vi "Processed_Bytes_To_CM_Packet.vi"(3 "error in (no error)":errorcluster, 4 "Processed Byte":u8[](array[numeric]), 5 "CM Packet In":T1) -> (0 "error out":errorcluster, 1 "CM Params":T5, 2 "CM Packet Out":T1)   [LabVIEW 2017]
uses:
  Controls/Packet/Packet.ctl
  Controls/Packet/Packet_Direction.ctl
  Controls/Packet/Packet_Type.ctl
  Controls/Packet/Packet_Priority.ctl
  Controls/Control Packets/CM_Param.ctl
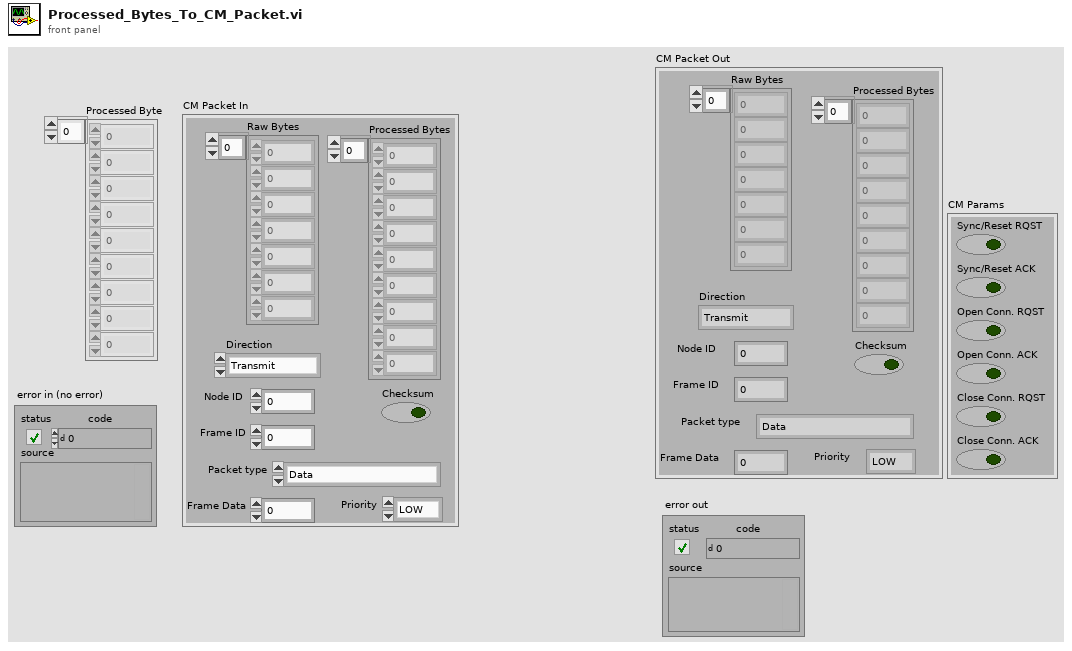
[diagram p1: front panel]
types:
  T1 = typedef "Packet.ctl" = cluster{"Raw Bytes":u8[], "Checksum":bool, "Direction":T2, "Processed Bytes":u8[], "Node ID":u8, "Packet type":T3, "Frame Data":u32, "Priority":T4, "Frame ID":u8}
  T2 = typedef "Packet_Direction.ctl" = enum16{"Transmit", "Receive", "Bidirectional"}
  T3 = typedef "Packet_Type.ctl" = enum16{"Data", "Connection Management", "Remote Request", "Error/Status"}
  T4 = typedef "Packet_Priority.ctl" = enum16{"LOW", "HIGH"}
  T5 = typedef "CM_Param.ctl" = cluster{"Sync/Reset RQST":bool, "Sync/Reset ACK":bool, "Open Conn. RQST":bool, "Open Conn. ACK":bool, "Close Conn. RQST":bool, "Close Conn. ACK":bool}
  T6 = typedef "ES_Param.ctl" = cluster{"Status Request":bool, "Status Ack.":bool, "Receiver Queue Status":enum16{"OK", "EMPTY", "FULL"}, "Network Error Status":enum16{"NONE", "CONNECTION_ALREADY_OPEN", "CONNECTION_ALREADY_CLOSED", "INVALID_FRAME_REQUEST"}, "Application Error Code":u16, "Receiver Queue Size":i32}
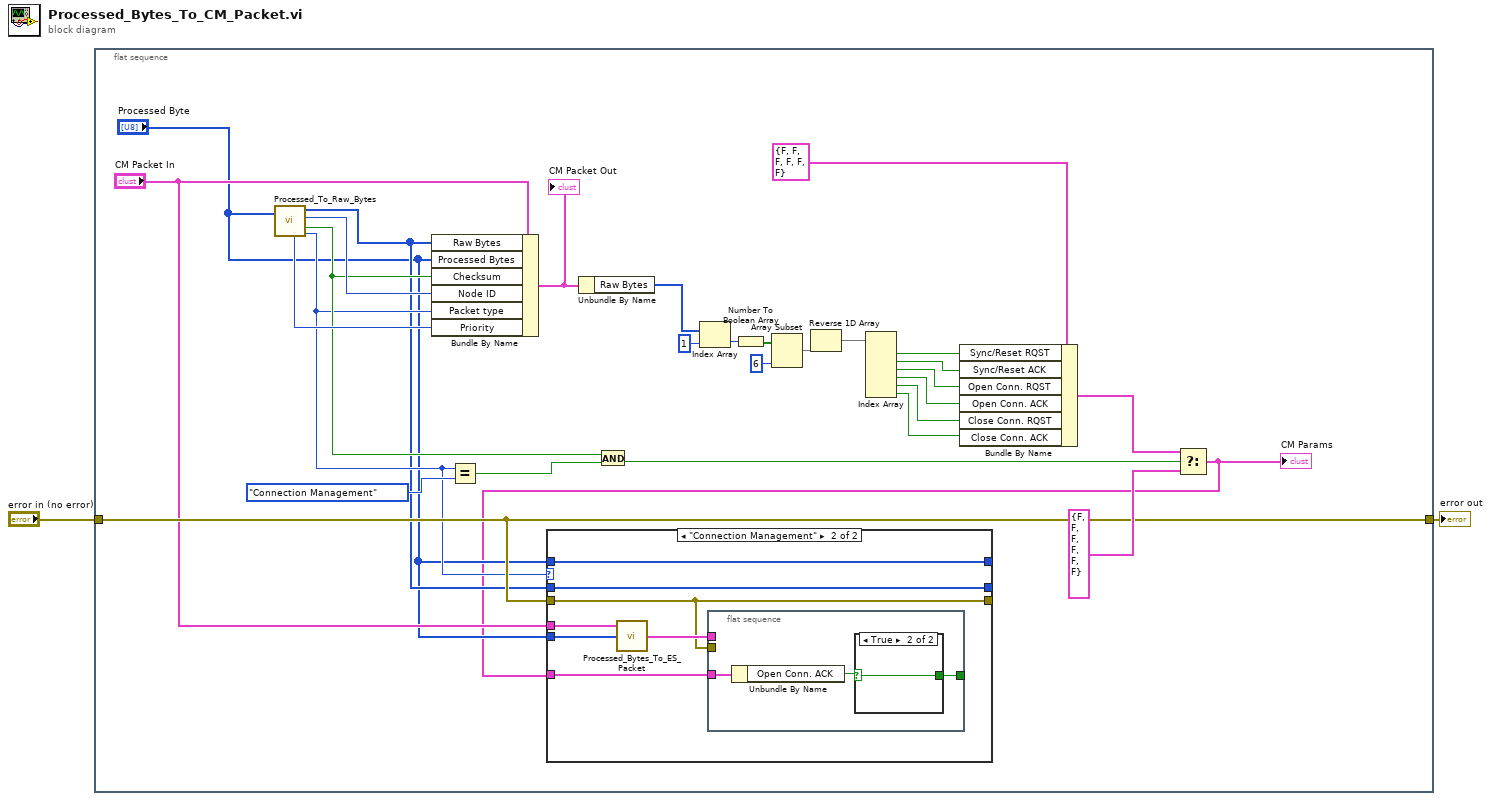
[diagram p0: block diagram]
diagram:
  n1 = flat-sequence {
    tunnel: "error in (no error)" -> [w8]
    tunnel: [w8] -> w1
    frame #0 {
      n2 = call "Processed_To_Raw_Bytes.vi"("Processed Bytes"="Processed Byte") -> ("Packet Type"=w7:T3, "Checksum"=w14:bool, "Node ID"=w31:u8, "Raw Bytes"=w6:u8[], "Priority"=w15:T4)  [unwired: 1 in]
      n3 = Bundle By Name(cluster="CM Packet In", "Raw Bytes"=w6, "Processed Bytes"="Processed Byte", "Checksum"=w14, "Node ID"=w31, "Packet type"=w7, "Priority"=w15) -> (w30:T1)
      "CM Packet Out" <- w30
      n4 = Equal?(x=w7, y=Packet_Type."Connection Management") -> (x = y?=w9:bool)
      n5 = Unbundle By Name(w30) -> ("Raw Bytes"=w29:u8[])
      n6 = And(x=w14, y=w9) -> (x .and. y?=w12:bool)
      n7 = Index Array(array=w29, index=1) -> (element=w27:u8)
      n8 = Number To Boolean Array(number=w27) -> (Boolean array=w18:bool[])
      n9 = Array Subset(array=w18, length=6) -> (w17:bool[])  [unwired: 1 in]
      n10 = Reverse 1D Array(array=w17) -> (reversed array=w25:bool[])
      n11 = Index Array(array=w25) -> (element #1=w24:bool, element #2=w23:bool, element #3=w22:bool, element #4=w21:bool, element #5=w20:bool, element #6=w19:bool)  [unwired: 6 in]
      n12 = Bundle By Name(cluster=T5 {"Sync/Reset RQST"=FALSE, "Sync/Reset ACK"=FALSE, "Open Conn. RQST"=FALSE, "Open Conn. ACK"=FALSE, "Close Conn. RQST"=FALSE, "Close Conn. ACK"=FALSE} ("Cluster"), "Sync/Reset RQST"=w24, "Sync/Reset ACK"=w23, "Open Conn. RQST"=w22, "Open Conn. ACK"=w21, "Close Conn. RQST"=w20, "Close Conn. ACK"=w19) -> (w11:T5)
      n13 = Select(t=w11, s=w12, f=T5 {"Sync/Reset RQST"=FALSE, "Sync/Reset ACK"=FALSE, "Open Conn. RQST"=FALSE, "Open Conn. ACK"=FALSE, "Close Conn. RQST"=FALSE, "Close Conn. ACK"=FALSE}) -> (s? t:f=w3:T5)
      "CM Params" <- w3
      n14 = case shown="\"Connection Management\"" w7 {
        tunnel: w8 -> [w34 w35]
        tunnel: [w34 w35] -> _
        tunnel: w6 -> [w33 w41]
        tunnel: [w33 w41] -> _
        tunnel: "Processed Byte" -> [w32 w40]
        tunnel: [w32 w40] -> _
        tunnel: "CM Packet In" -> [_ w39]
        tunnel: "Processed Byte" -> [_ w38]
        tunnel: w3 -> [_ w36]
        frame "Data", Default {
        }
        frame "Connection Management" {
          n15 = call "Processed_Bytes_To_ES_Packet.vi"("Processed_Bytes"=w38, "ES Packet In"=w39) -> ("ES Param Out"=w37:T6)  [unwired: 1 in, 2 out]
          n16 = flat-sequence {
            tunnel: w37 -> [_]
            tunnel: w36 -> [w44]
            tunnel: w35 -> [_]
            tunnel: [w42] -> _
            frame #0 {
              n17 = Unbundle By Name(w44) -> ("Open Conn. ACK"=w43:bool)
              n18 = case shown="True" w43 {
                selector: w43 -> [w45 w46]
                tunnel: [w45 w46] -> w42
                frame False {
                }
                frame True {
                }
              }
            }
          }
        }
      }
    }
  }
  "error out" <- w1
